vi "action.vi"(0 "MoAgSy_Visitor in":refnum<class "MoAgSy_Visitor.lvclass">, 2 "HGF_Visitable":refnum<class "HGF_Visitable.lvclass">, 5 "error in (no error)":errorcluster) -> (14 "MoAgSy_Visitor out":refnum<class "MoAgSy_Visitor.lvclass">, 16 "dup HGF_Visitable":refnum<class "HGF_Visitable.lvclass">, 19 "error out":errorcluster)   [LabVIEW 2009, in "MoAgSy_Base.lvlib" / "MoAgSy_Visitor.lvclass"]
doc: "This is a dynamic dispatch VI that is called from Visitor.visit(). It will call member VIs of Visitable to perform the requested action which means: calling public methods of Visitable child class.\n\n<B>Hint:</B> This method is abstract and need to be implemented by child classes."
uses:
  MoAgSy_Visitor.lvclass
  HGF_BaseClasses/HGF_Visitable/HGF_Visitable.lvclass
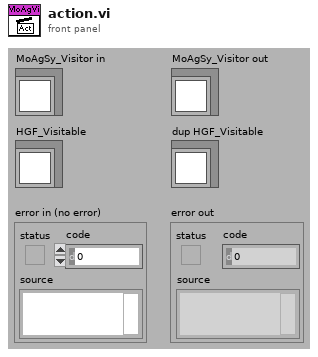
[diagram p1: front panel]
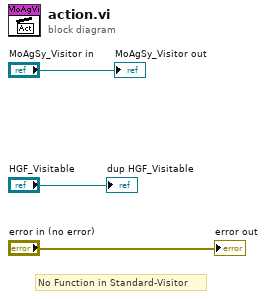
[diagram p0: block diagram]
diagram:
  # "No Function in Standard-Visitor"
  "error out" <- "error in (no error)"
  "MoAgSy_Visitor out" <- "MoAgSy_Visitor in"
  "dup HGF_Visitable" <- "HGF_Visitable"
